vi "Test Open Read Close Vorbis.vi"(8 "error in (no error)":errorcluster) -> (0 "error out":errorcluster, 3 "Pass?":bool)   [LabVIEW 2020]
uses:
  G-Audio/Audio Files/Polymorphic VIs/Get Audio File Info (Path).vi
  G-Audio/Audio Files/Polymorphic VIs/Open Audio File Read (Path).vi
  be8f713a-8f42-4c3e-86c0-705fec61fa9c.vi
  1bc2927e-03b6-4d5d-acbf-232c83f81b01.vi
  G-Audio/Private/Path To UTF-8 String.vi
  G-Audio/Audio Files/Private/Get Audio File Info (Core).vi
  G-Audio/Audio Files/Private/Open Audio File Read (Core).vi
  G-Audio/Private/Get Basic Audio File Info.vi
  G-Audio/Private/Result To Error.vi
  be8f713a-8f42-4c3e-86c0-705fec61fa9c.vi/779dfdfd-1b42-4cf4-8001-66d3dd167625.vi
  be8f713a-8f42-4c3e-86c0-705fec61fa9c.vi/55d550d4-9624-414e-aebd-6e02b5081896.vi
  G-Audio/Private/Audio File Refnum To Value.vi
  G-Audio/Private/Value To Audio File Refnum.vi
  be8f713a-8f42-4c3e-86c0-705fec61fa9c.vi/55d550d4-9624-414e-aebd-6e02b5081896.vi/4b7b629c-2e91-4160-9820-a26af8f6e677.vi
  <vilib>/sound2/lvsound2.llb/Sound File Read Open.vi
  <vilib>/sound2/lvsound2.llb/Sound File Info (refnum).vi
  <vilib>/sound2/lvsound2.llb/Sound File Read (I16).vi
  <vilib>/Utility/error.llb/Error Cluster From Error Code.vi
  <vilib>/Utility/Data Type/Get Numeric Information.vi
  G-Audio/G-Audio.lvlib
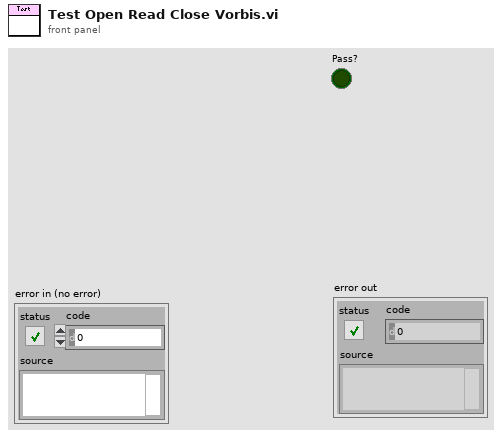
[diagram p1: front panel]
types:
  T1 = typedef "G-Audio.lvlib/Audio File Info.ctl" = cluster{"Sample Rate (Hz)":u32, "Channels":u32, "Bit Depth":u32}
  T2 = typedef "Sound File Refnum.ctl" = refnum<file>
  T3 = typedef "Sound Data Format.ctl" = cluster{"sample rate (S/s)":dbl, "number of channels":i32, "bits per sample":i32}
  T4 = typedef "G-Audio.lvlib/Audio File Refnum.ctl" = refnum<file>
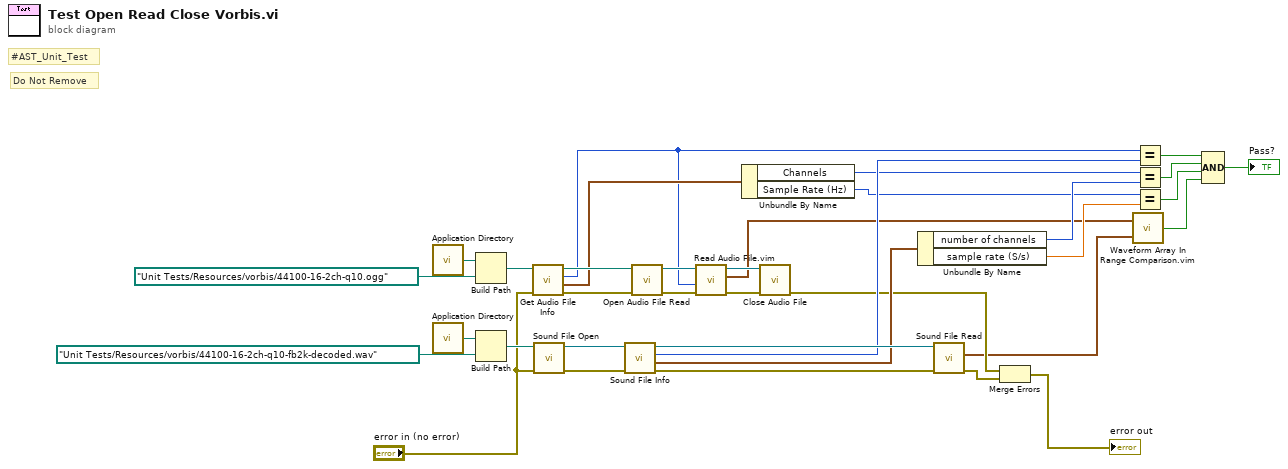
[diagram p0: block diagram]
diagram:
  # "Do Not Remove"
  # "#AST_Unit_Test"
  n1 = call <vilib>:"Application Directory.vi"() -> ("Application Directory"=w6:path)
  n2 = call <vilib>:"Application Directory.vi"() -> ("Application Directory"=w35:path)
  n3 = Build Path(base path=w6, name or relative path=path "Unit Tests/Resources/vorbis/44100-16-2ch-q10.ogg" ("Path")) -> (appended path=w4:path)
  n4 = Build Path(base path=w35, name or relative path=path "Unit Tests/Resources/vorbis/44100-16-2ch-q10-fb2k-decoded.wav" ("Path")) -> (appended path=w34:path)
  n5 = call-poly "Get Audio File Info.vi"("error in (no error)"="error in (no error)", "Path In"=w4) -> ("error out"=w3:errorcluster, "Audio File Info"=w16:T1, "PCM Frame Length"=w1:u64, "Path Out"=w18:path)  [unwired: 5 in, 1 out]
  n6 = call-poly <vilib>:"Sound File Open.vi"("error in (no error)"="error in (no error)", "path"=w34) -> ("error out"=w23:errorcluster, "sound file refnum"=w32:T2)  [unwired: 8 in]
  n7 = call-poly <vilib>:"Sound File Info.vi"("error in (no error)"=w23, "sound file refnum"=w32) -> ("error out"=w22:errorcluster, "sound format"=w27:T3, "total number of samples/ch"=w28:u32, "sound file refnum out"=w31:T2)  [unwired: 6 in]
  n8 = call-poly "Open Audio File Read.vi"("error in (no error)"=w3, "Path"=w18) -> ("error out"=w13:errorcluster, "Audio File Refnum"=w17:T4)  [unwired: 8 in]
  n9 = call "Read Audio File.vim"("error in (no error)"=w13, "Frames To Read"=w1, "Audio File Refnum In"=w17) -> ("error out"=w11:errorcluster, "Audio Data"=w8:waveform(i16)[], "Audio File Refnum Out"=w12:T4)  [unwired: 4 in, 2 out]
  n10 = Unbundle By Name(w16) -> ("Channels"=w15:u32, "Sample Rate (Hz)"=w14:u32)
  n11 = call "Close Audio File.vi"("error in (no error)"=w11, "Audio File Refnum In"=w12) -> ("error out"=w10:errorcluster)  [unwired: 9 in]
  n12 = Unbundle By Name(w27) -> ("number of channels"=w26:i32, "sample rate (S/s)"=w19:dbl)
  n13 = call-poly <vilib>:"Sound File Read.vi"("error in (no error)"=w22, "sound file refnum"=w31) -> ("error out"=w21:errorcluster, "data"=w9:waveform(i16)[])  [unwired: 5 in, 3 out]
  n14 = Merge Errors(w10, w21) -> (→"error out":errorcluster)
  n15 = call "Waveform Array In Range Comparison.vim"("Expected Value"=w9, "Resulting Value"=w8) -> ("Comparison Result"=w7:bool)
  n16 = Equal?(x=w1, y=w28) -> (x = y?=w30:bool)
  n17 = Equal?(x=w15, y=w26) -> (x = y?=w25:bool)
  n18 = Equal?(x=w14, y=w19) -> (x = y?=w24:bool)
  n19 = Compound Arithmetic op=AND(w30, w25, w24, w7) -> (→"Pass?":bool)
